vi "Generate Unique Header.vi"(8 "error in":errorcluster, 11 "Vaisala Data in":refnum<class "Vaisala Data.lvclass">) -> (0 "error out":errorcluster, 2 "Header":string[](array[string]), 3 "Vaisala Data out":refnum<class "Vaisala Data.lvclass">)   [LabVIEW 2014, in "Vaisala Library.lvlib" / "Vaisala Data.lvclass"]
uses:
  Vaisala Data.lvclass
  reusable/Data/Data.lvlibp/Read Data ID.vi
  reusable/Data/Data.lvlibp/Data.lvclass
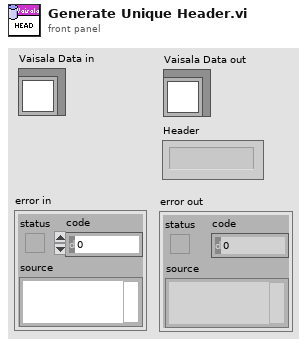
[diagram p1: front panel]
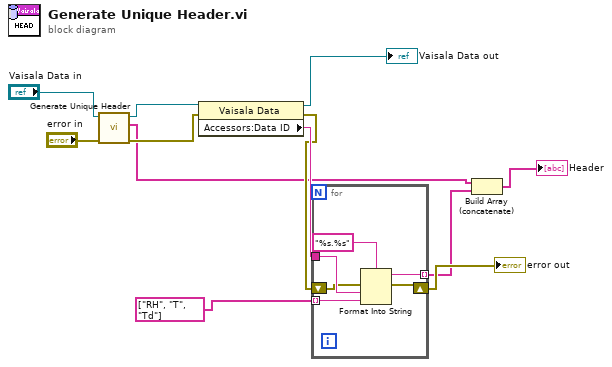
[diagram p0: block diagram]
diagram:
  n1 = call-parent "Generate Unique Header.vi"("error in"="error in", "Data in"="Vaisala Data in") -> ("error out"=w8:errorcluster, "Header"=w3:string[], "Data out"=w10:refnum<class "Vaisala Data.lvclass">)  [unwired: 7 in]
  n2 = property class="Vaisala Data"(reference=w10, error in=w8) -> (reference out=→"Vaisala Data out":refnum<class "Vaisala Data.lvclass">, error out=w5:errorcluster, "Accessors:Data ID"=w7:string)
  n3 = for {
    tunnel: w7 -> [w18]
    tunnel: [w16] -> w2 mode=indexing
    tunnel: string[] ["RH", "T", "Td"] -> [w15] mode=indexing
    shift-right: [w14] -> w4
    shift-left: w5 -> [w13]
    n4 = Format Into String(format string="%s.%s", error in=w13, w18, w15) -> (resulting string=w16:string, error out=w14:errorcluster)  [unwired: 1 in]
  }
  "error out" <- w4
  n5 = Build Array (concatenate)(w3, w2) -> (→"Header":string[])
